vi "Write Data.vi"(8 "error in (no error)":errorcluster, 9 "Publication Time":timestamp, 10 "Value":variant, 11 "BooleanTextBinding in":refnum<class "FormattedStringBinding.lvclass">) -> (0 "error out":errorcluster, 3 "BooleanTextBinding out":refnum<class "FormattedStringBinding.lvclass">)   [LabVIEW 2017, in "Transport.lvlib" / "FormattedStringBinding.lvclass"]
doc: "<License>\nCopyright © 2017 Composed Systems, LLC | All rights reserved\nwww.composed.io\n\nAuthor: Ethan Stern <ethan.stern@composed.io>\n\nThis software is provided \"AS IS\" WITHOUT WARRANTIES, either express or implied, AND IS FOR EDUCATIONAL PURPOSES ONLY.\n</License>"
uses:
  FormattedStringBinding.lvclass
  FormattedStringBinding.lvclass/FormattedStringBinding.ctl
  <vilib>/Utility/error.llb/Error Cluster From Error Code.vi
  <vilib>/ErrorRing/Error Ring.xnode
  <vilib>/Utility/Data Type/NI_Data Type.lvlib
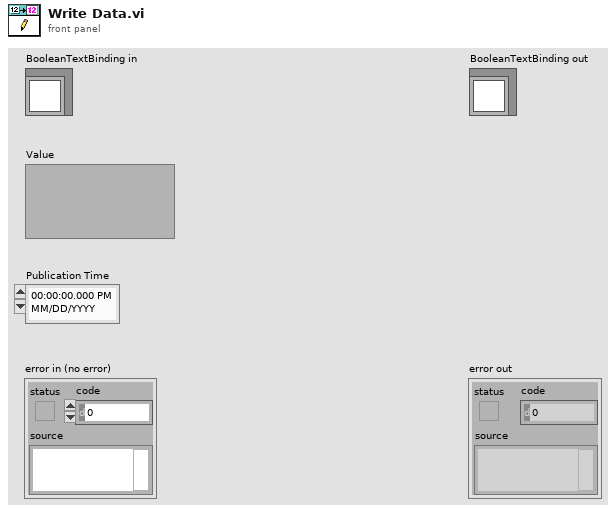
[diagram p1: front panel]
types:
  T1 = typedef "NI_Data Type.lvlib/Data Type.ctl" = enum8{"Invalid Type", "Void", "I8", "I16", "I32", "I64", "U8", "U16", "U32", "U64", "Single Float", "Double Float", "Extended Float", "Single Complex", "Double Complex", "Extended Complex", "Enum U8", "Enum U16", "Enum U32", "Enum U64", "Single Float With Unit", "Double Float With Unit", "Extended Float With Unit", "Single Complex with Unit", "Double Complex with Unit", "Extended Complex with Unit", "Boolean", "String", "Path", "Picture", "Tag", "Array", "Cluster", "Variant", "LV Variant", "Waveform", "Timestamp", "Digital Waveform", "Digital Data", "ExpressData", "Refnum", "External Data", "VI", "Poly VI", "LabVIEW Class Instance", "Fixed Point"}
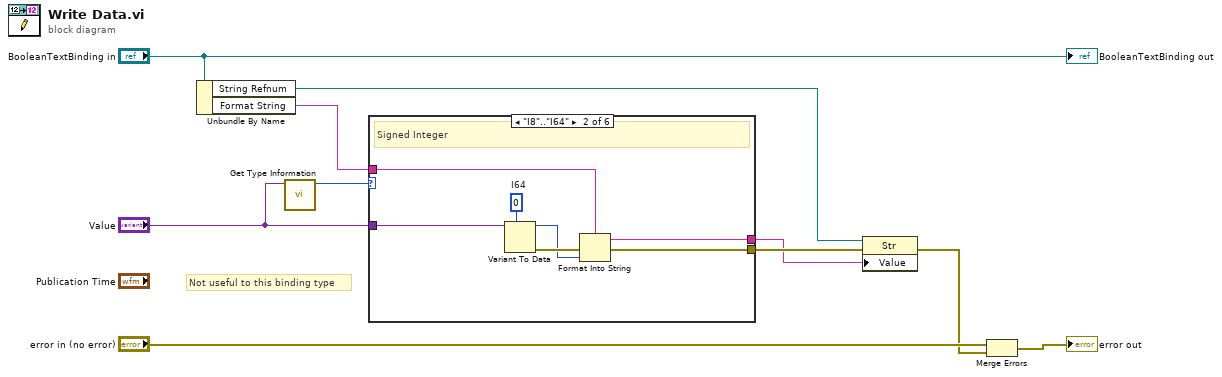
[diagram p0: block diagram]
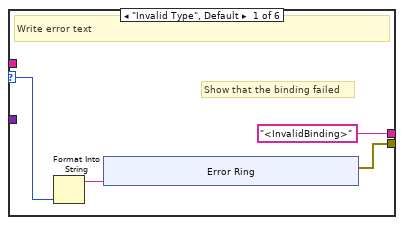
[diagram p2: hidden frame]
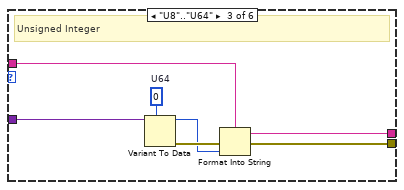
[diagram p3: hidden frame]
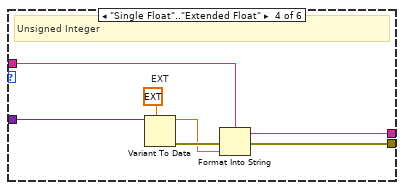
[diagram p4: hidden frame]
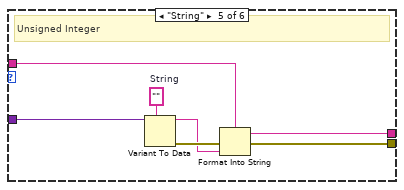
[diagram p5: hidden frame]
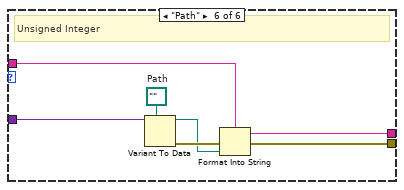
[diagram p6: hidden frame]
diagram:
  # "Not useful to this binding type"
  n1 = Unbundle By Name("BooleanTextBinding in") -> ("String Refnum"=w7:refnum<vi>, "Format String"=w5:string)
  n2 = call <vilib>:"Get Type Information.vi"("Variant"="Value") -> ("Type"=w1:T1)  [unwired: 6 in, 4 out]
  n3 = case shown="\"I8\"..\"I64\"" w1 {
    selector: w1 -> [w12 _ _ _ _ _]
    tunnel: "Value" -> [_ w28 w35 w42 w49 w56]
    tunnel: w5 -> [_ w27 w34 w41 w48 w55]
    tunnel: [w13 w25 w32 w39 w46 w53] -> w4
    tunnel: ["<InvalidBinding>" w24 w31 w38 w45 w52] -> w3
    frame "Invalid Type", Default {
      # "Show that the binding failed"
      # "Write error text"
      n4 = Format Into String(w12) -> (resulting string=w11:string)  [unwired: 3 in, 1 out]
      n5 = xnode "Error Ring"("parameter 0"=w11) -> ("error out"=w13:errorcluster)
    }
    frame "I8".."I64" {
      w22 = i64 0  # I64
      # "Signed Integer"
      n6 = Variant To Data(type=w22, Variant=w28) -> (data=w23:i64, error out=w26:errorcluster)  [unwired: 1 in]
      n7 = Format Into String(format string=w27, error in=w26, w23) -> (resulting string=w24:string, error out=w25:errorcluster)  [unwired: 1 in]
    }
    frame "U8".."U64" {
      w29 = u64 0  # U64
      # "Unsigned Integer"
      n8 = Variant To Data(type=w29, Variant=w35) -> (data=w30:u64, error out=w33:errorcluster)  [unwired: 1 in]
      n9 = Format Into String(format string=w34, error in=w33, w30) -> (resulting string=w31:string, error out=w32:errorcluster)  [unwired: 1 in]
    }
    frame "Single Float".."Extended Float" {
      w36 = ext 0.0  # EXT
      # "Unsigned Integer"
      n10 = Variant To Data(type=w36, Variant=w42) -> (data=w37:ext, error out=w40:errorcluster)  [unwired: 1 in]
      n11 = Format Into String(format string=w41, error in=w40, w37) -> (resulting string=w38:string, error out=w39:errorcluster)  [unwired: 1 in]
    }
    frame "String" {
      w43 = ""  # String
      # "Unsigned Integer"
      n12 = Variant To Data(type=w43, Variant=w49) -> (data=w44:string, error out=w47:errorcluster)  [unwired: 1 in]
      n13 = Format Into String(format string=w48, error in=w47, w44) -> (resulting string=w45:string, error out=w46:errorcluster)  [unwired: 1 in]
    }
    frame "Path" {
      w50 = path ""  # Path
      # "Unsigned Integer"
      n14 = Variant To Data(type=w50, Variant=w56) -> (data=w51:path, error out=w54:errorcluster)  [unwired: 1 in]
      n15 = Format Into String(format string=w55, error in=w54, w51) -> (resulting string=w52:string, error out=w53:errorcluster)  [unwired: 1 in]
    }
  }
  n16 = property class="Str"(reference=w7, error in=w4, "Value"=w3) -> (error out=w6:errorcluster)  [unwired: 1 out]
  n17 = Merge Errors("error in (no error)", w6) -> (→"error out":errorcluster)
  "BooleanTextBinding out" <- "BooleanTextBinding in"
